vi "Acquire Body Index Image.vi"() -> ()   [LabVIEW 2014, in "LVH-KinectOne.lvlib"]
doc: "This example demonstrates how to acquire a Body Index frame from the Microsoft Kinect One."
uses:
  vi.lib/LabVIEW Hacker/KinectOne/LVH-KinectOne.lvlib
  vi.lib/LabVIEW Hacker/KinectOne/Private/Initialize Image [Body Index].vi
  vi.lib/LabVIEW Hacker/KinectOne/Private/kinectRead [BodyIndexFrame].vi
panel:
  in  "Stop Button":bool
  out "Body Index Image":T1(plugin-control)
  # "LVH Interface for Kinect One \nAcquire Body Index Image Example\n\nThis example demonstrates how to acquire body index images from the Kinect One.\n\n1. Make sure you have the Kinect SDK 2.0 installed.\n2. Connect the Kinect sensor to the computer via USB.\n3. Click the Run button.\n4. Stand in front of the Kinect sensor.\n\nHave feedback or need help?  Visit the LabVIEW Hacker forums at www.labviewhacker.com/forums/kinect"
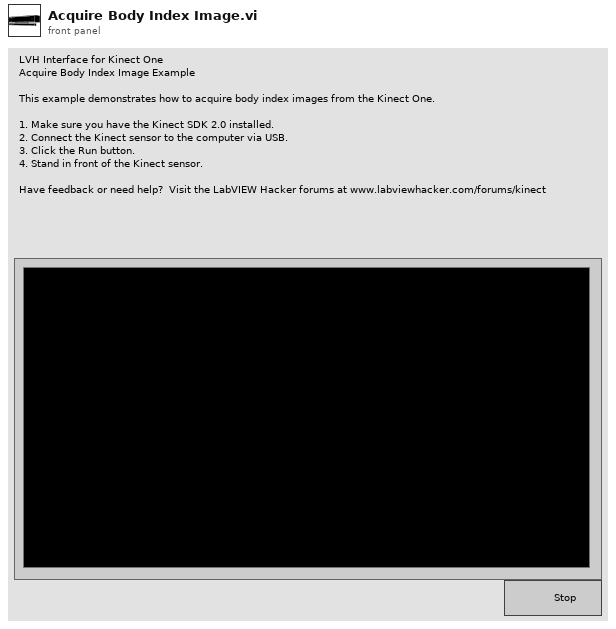
[diagram p1: front panel]
types:
  T1 = typedef "IMAQ Image.ctl" = refnum<image>
  T2 = typedef "LVH-KinectOne.lvlib/KinectSensor References.ctl" = cluster{"KinectSensor":refnum<k24>, "MultiSourceFrameReader":refnum<k24>, "BodyFrameDataInterface":refnum<k24>}
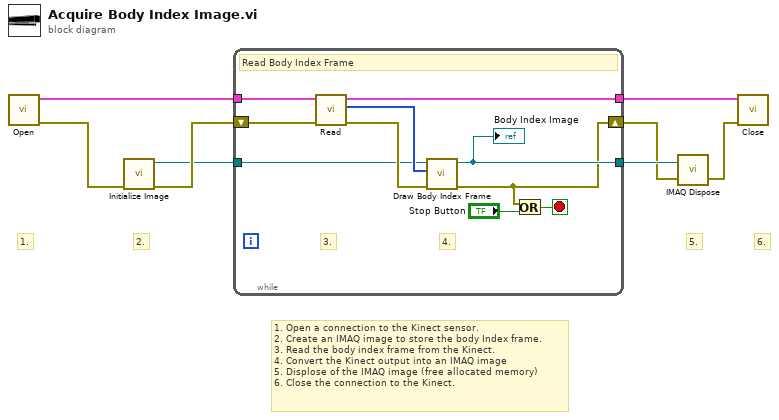
[diagram p0: block diagram]
diagram:
  # "1. Open a connection to the Kinect sensor.\n2. Create an IMAQ image to store the body Index frame.\n3. Read the body index frame from the Kinect.\n4. Convert the Kinect output into an IMAQ image\n5. Displose of the IMAQ image (free allocated memory)\n6. Close the connection to the Kinect."
  # "6."
  # "5."
  # "2."
  # "1."
  n1 = call "Open.vi"() -> ("Error Out"=w3:errorcluster, "KinectSensor References out"=w4:T2)  [unwired: 10 in]
  n2 = call-poly "Initialize Image.vi"("Error In"=w3) -> ("Error Out"=w2:errorcluster, "Body Index Image"=w1:T1)  [unwired: 9 in]
  n3 = while {
    tunnel: w4 -> [w18]
    tunnel: [w14] -> w8
    shift-right: [w11] -> w6
    shift-left: w2 -> [w17]
    tunnel: w1 -> [w13]
    tunnel: [w12] -> w7
    stop <- w10 stop-if-true
    # "4."
    # "3."
    # "Read Body Index Frame"
    n4 = call-poly "Read.vi"("Error In"=w17, "KinectSensor References in"=w18) -> ("Error Out"=w16:errorcluster, "frameData"=w15:u8[], "KinectSensor References out"=w14:T2)  [unwired: 7 in]
    n5 = call "Draw Body Index Frame.vi"("Error In"=w16, "Byte Array"=w15, "Image"=w13) -> ("Error Out"=w11:errorcluster, "Image Out"=w12:T1)  [unwired: 7 in]
    "Body Index Image" <- w12
    n6 = Or(x=w11, y="Stop Button") -> (x .or. y?=w10:bool)
  }
  n7 = call "IMAQ Dispose"("Image"=w7, "error in (no error)"=w6) -> ("error out"=w5:errorcluster)  [unwired: 4 in]
  n8 = call "Close.vi"("Error In"=w5, "KinectSensor References"=w8) -> ()  [unwired: 9 in, 1 out]
